vi "MSE.vi"(2 "X Values":dbl[](array[numeric]) format="%0.2f", 3 "Y Values":dbl[](array[numeric]) format="%0.2f") -> (0 "error":i32, 1 "mse":dbl format="%0.2f")   [LabVIEW 2020, in "NI_AALPro.lvlib"]
doc: "Computes the mean square error (<B>mse</B>) of the input sequences <B>X Values</B> and <B>Y Values</B>."
uses:
  <vilib>/Analysis/NI_AALPro.lvlib
  <resource>/lvanlys.dll
panel:
  # "Mean Square Error"
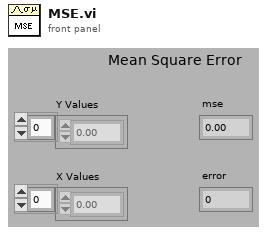
[diagram p1: front panel]
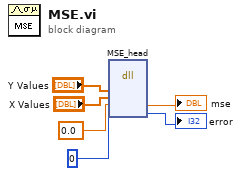
[diagram p0: block diagram]
diagram:
  n1 = dll-call lib="e:/builds/penguin/labview/branches/2020/dev/dist/resource/lvanlys.*" fn="MSE_head"("Y Values"="Y Values", "X Values"="X Values", "output param"=0.0, "output param"=0) -> ("output param"=→"mse":dbl, "output param"=→"error":i32)  [unwired: 6 in, 2 out]
